vi "changeConfiguration.vi"(8 "error in (no error)":errorcluster, 10 "configuration":string, 11 "StartSAL.lvclass in":refnum<class "StartSAL.lvclass">) -> (0 "error out":errorcluster, 3 "StartSAL.lvclass out":refnum<class "StartSAL.lvclass">)   [LabVIEW 2016, in "StartSAL.lvclass"]
uses:
  StartSAL.lvclass
  StartSAL.lvclass/StartSAL.ctl
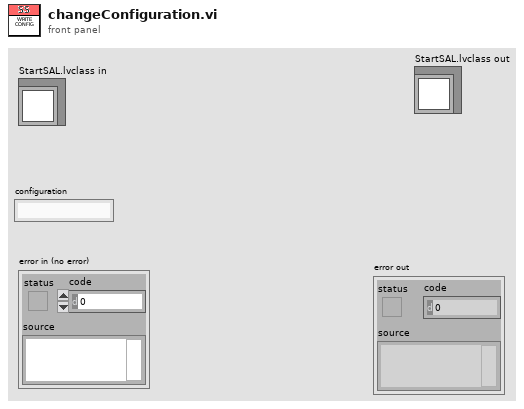
[diagram p1: front panel]
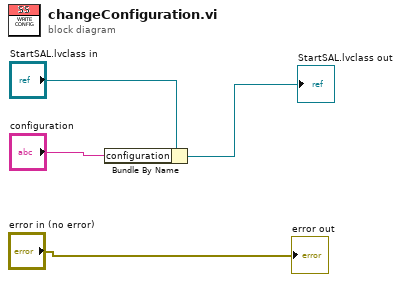
[diagram p0: block diagram]
diagram:
  n1 = Bundle By Name(cluster="StartSAL.lvclass in", "configuration"="configuration") -> (→"StartSAL.lvclass out":refnum<class "StartSAL.lvclass">)
  "error out" <- "error in (no error)"
